vi "show_MagFieldTables.vi"() -> ()   [LabVIEW 2013]
uses:
  Classes/MagFieldTable/MagFieldTable.lvclass
panel:
  out "subarray":string[](array[string])
  out "name":string
  in  "index to read":dbl
  out "Array Size":i32
  out "Table Control":string[][](table)
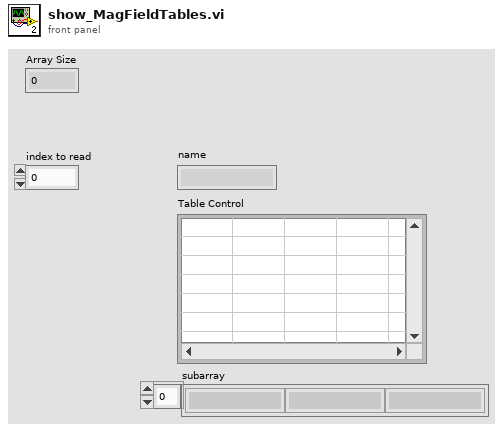
[diagram p1: front panel]
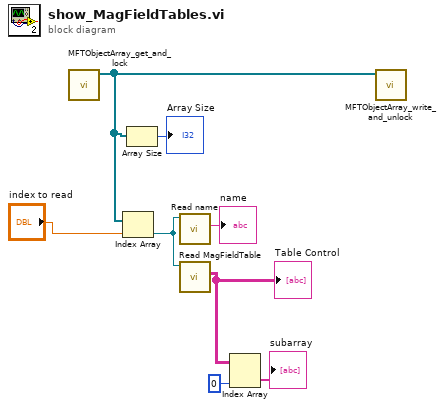
[diagram p0: block diagram]
diagram:
  n1 = call "MFTObjectArray_get_and_lock.vi"() -> ("MFTObjects"=w7:refnum<class "MagFieldTable.lvclass">[])  [unwired: 10 in, 1 out]
  n2 = Index Array(array=w7, index="index to read") -> (element=w6:refnum<class "MagFieldTable.lvclass">)
  n3 = Array Size(array=w7) -> (size(s)=→"Array Size":i32)
  n4 = call-dynamic "Read name.vi"("MagFieldTable in"=w6) -> ("name"=→"name":string)  [unwired: 8 in, 2 out]
  n5 = call-dynamic "Read MagFieldTable.vi"("MagFieldTable in"=w6) -> ("MagFieldTable"=w3:string[][])  [unwired: 8 in, 2 out]
  "Table Control" <- w3
  n6 = Index Array(array=w3, index (col)=0 ("disabled index (col)")) -> (element=→"subarray":string[])  [unwired: 1 in]
  n7 = call "MFTObjectArray_write_and_unlock.vi"("MFTObjects"=w7) -> ()  [unwired: 10 in, 1 out]
